vi "CheckPhaseShift.vi"(11 "3-phase phase degree":dbl[](array[numeric])) -> (3 "all 120-degree shift?":bool)   [LabVIEW 2017, in "McsaAnalysisLowRate.lvlib"]
uses:
  <vilib>/addons/InsightCM/Devices/Shared/Mcsa/McsaAnalysisLowRate/McsaAnalysisLowRate.lvlib
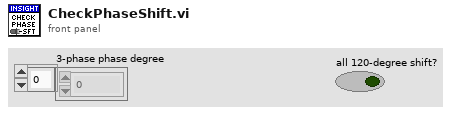
[diagram p1: front panel]
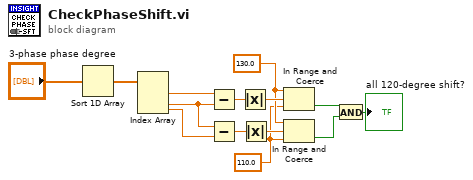
[diagram p0: block diagram]
diagram:
  w4 = 110.0 ("upper limit")
  w5 = 130.0 ("upper limit")
  n1 = Sort 1D Array(array="3-phase phase degree") -> (sorted array=w13:dbl[])
  n2 = Index Array(array=w13) -> (element #1=w10:dbl, element #2=w11:dbl, element #3=w12:dbl)  [unwired: 3 in]
  n3 = Subtract(x=w10, y=w11) -> (x-y=w9:dbl)
  n4 = Subtract(x=w11, y=w12) -> (x-y=w8:dbl)
  n5 = Absolute Value(x=w9) -> (abs(x)=w7:dbl)
  n6 = Absolute Value(x=w8) -> (abs(x)=w6:dbl)
  n7 = In Range and Coerce(upper limit=w5, x=w7, lower limit=w4) -> (In Range?=w3:bool)  [unwired: 1 out]
  n8 = In Range and Coerce(upper limit=w5, x=w6, lower limit=w4) -> (In Range?=w2:bool)  [unwired: 1 out]
  n9 = And(x=w3, y=w2) -> (x .and. y?=→"all 120-degree shift?":bool)
